vi "Method No Arguments.vi"(8 "error in (no error)":errorcluster, 11 "Mock In":refnum<class "Test Interface Pure Mock.lvclass">) -> (0 "error out":errorcluster, 3 "Mock Out":refnum<class "Test Interface Pure Mock.lvclass">)   [LabVIEW 2020, in "Test Interface Pure Mock.lvclass"]
uses:
  Test Interface Pure Mock.lvclass
  C:/git/astemes-lmock/source/Framework/Pure Mock/Pure Mock.lvclass
  source/Framework/Pure Mock/Pure Mock.lvclass/Pure Mock.ctl
  source/Framework/VI Server VI Call/Create.vi
  source/Core/Expectation/Expectation.lvclass
  source/Framework/Pure Mock/Pure Mock.lvclass
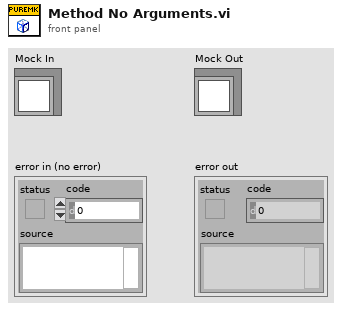
[diagram p1: front panel]
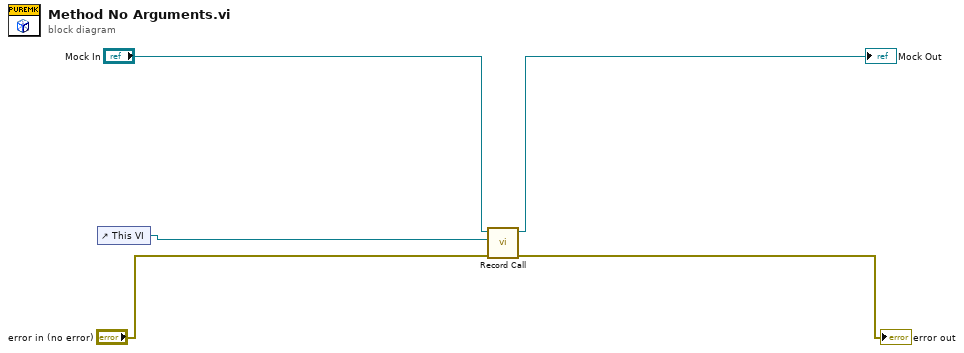
[diagram p0: block diagram]
diagram:
  n1 = control-ref of="This VI"() -> (w5:refnum<vi>)
  n2 = call "Record Call.vi"("error in (no error)"="error in (no error)", "This VI"=w5, "Mock In"="Mock In") -> ("error out"=→"error out":errorcluster, "Mock Out"=→"Mock Out":refnum<class "Test Interface Pure Mock.lvclass">)  [unwired: 7 in]
